vi "Control, Center Y on Panel.vi"(0 "error in":errorcluster, 2 "Ctl ref":refnum<vi>, 3 "VI ref":refnum<vi>) -> (7 "error out":errorcluster, 9 "Ctl ref dup":refnum<vi>, 10 "VI ref dup":refnum<vi>)   [LabVIEW 2010]
doc: "This function centers a GUI control along the vertical axis (Y) of a panel."
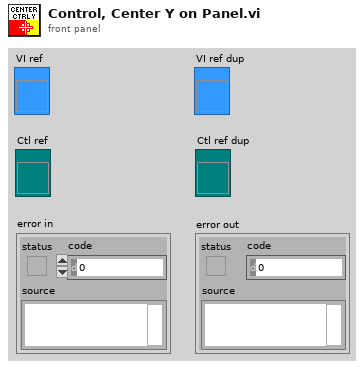
[diagram p1: front panel]
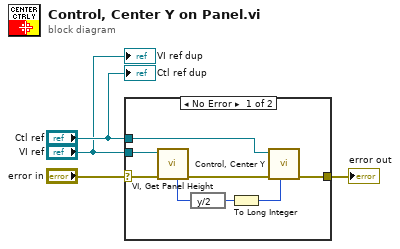
[diagram p0: block diagram]
diagram:
  n1 = case shown="No Error" "error in" {
    selector: "error in" -> [w12 w13]
    tunnel: [w10 w13] -> w4
    tunnel: "Ctl ref" -> [w5 _]
    tunnel: "VI ref" -> [w6 _]
    frame No Error {
      n2 = call "VI, Get Panel Height.vi"("error in"=w12, "VI ref"=w6) -> ("error out"=w11:errorcluster, "height"=w9:i16)  [unwired: 5 in, 1 out]
      n3 = expression code="y/2"(w9) -> (w8:i16)
      n4 = To Long Integer(number=w8) -> (32bit integer=w7:i32)
      n5 = call "Control, Center Y.vi"("error in"=w11, "Ctl ref"=w5, "Y (0)"=w7) -> ("error out"=w10:errorcluster)  [unwired: 6 in, 1 out]
    }
    frame Error {
    }
  }
  "error out" <- w4
  "Ctl ref dup" <- "Ctl ref"
  "VI ref dup" <- "VI ref"
